vi "Menu 1.vi"() -> ()   [LabVIEW 2015]
panel:
  in  "stop":bool
  in  "Change menu":bool
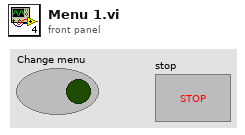
[diagram p1: front panel]
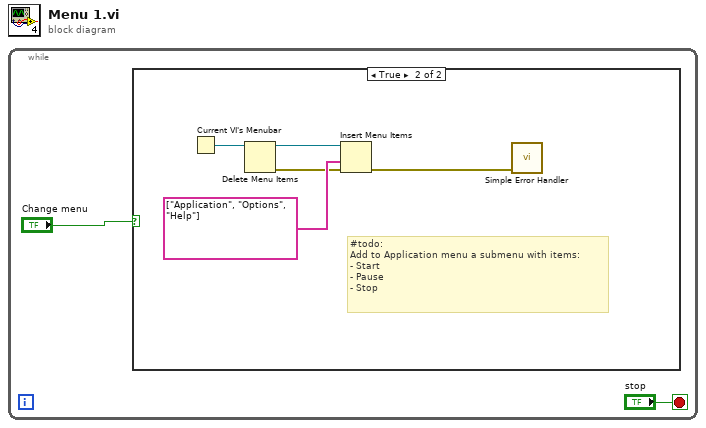
[diagram p0: block diagram]
diagram:
  n1 = while {
    stop <- "stop" stop-if-true
    n2 = case shown="True" "Change menu" {
      frame False {
      }
      frame True {
        # "#todo:\nAdd to Application menu a submenu with items:\n- Start\n- Pause\n- Stop"
        n3 = Current VI's Menubar() -> (w5:refnum<k9>)
        n4 = Delete Menu Items(9:w5) -> (0:w4:errorcluster, 3:w6:refnum<k9>)  [unwired: 3 in]
        n5 = Insert Menu Items(6:w4, 7:string[] ["Application", "Options", "Help"] ("L10n_item tags 1"), 9:w6) -> (0:w3:errorcluster)  [unwired: 3 in, 2 out]
        n6 = call <vilib>:"Simple Error Handler.vi"("error in (no error)"=w3) -> ()  [unwired: 4 in, 5 out]
      }
    }
  }
